vi "avoidDisturbAttackerShoot.vi"(1 "CalculatedFollowAttackerPosition":dbl[](array[numeric]), 4 "AttackingOurSelves":bool=TRUE, 5 "Game":refnum<class "Game.lvclass">, 6 "FollowAttackerPosition(FA)":dbl[](array[numeric]), 7 "field_length":i32, 8 "error in (no error)":errorcluster, 9 "AttackerPosition(AT)":dbl[](array[numeric]), 10 "Yball":dbl, 11 "FollowAttackerSkill in":refnum<class "FollowAttackerSkill.lvclass">) -> (0 "error out":errorcluster, 2 "FollowAttackerCorrectedPosition":dbl[](array[numeric]), 3 "FollowAttackerSkill out":refnum<class "FollowAttackerSkill.lvclass">)   [LabVIEW 2020, in "FollowAttackerSkill.lvclass"]
uses:
  FollowAttackerSkill.lvclass
  Game_class/Game.lvclass
  Game_class/Game.lvclass/Game.ctl
  Game_class/Read FieldRef.vi
  Game_class/Read Utilities.lvclass.vi
  Field_class/Field.lvclass
  Utilities_class/Utilities.lvclass
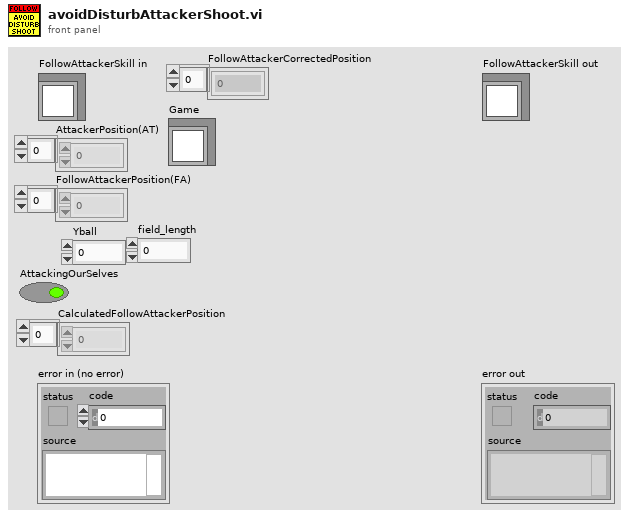
[diagram p1: front panel]
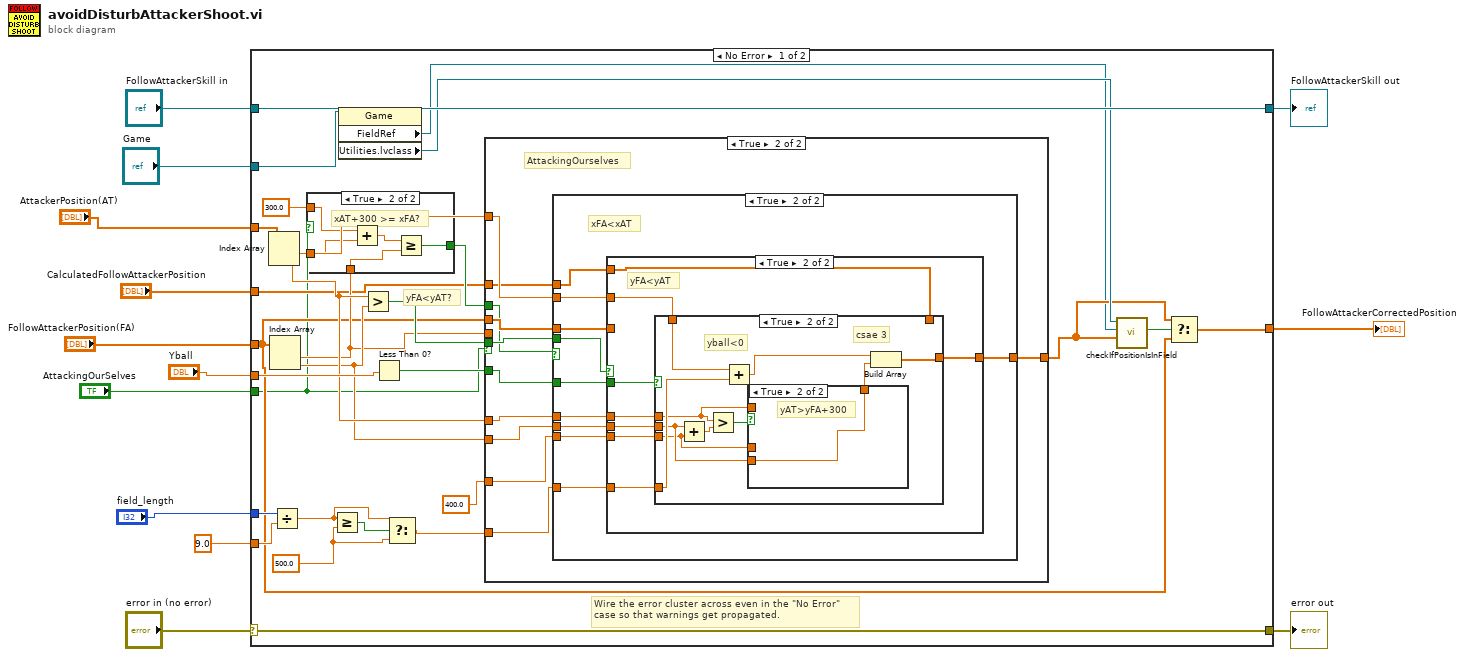
[diagram p0: block diagram]
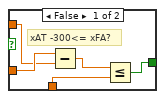
[diagram p2: hidden frame]
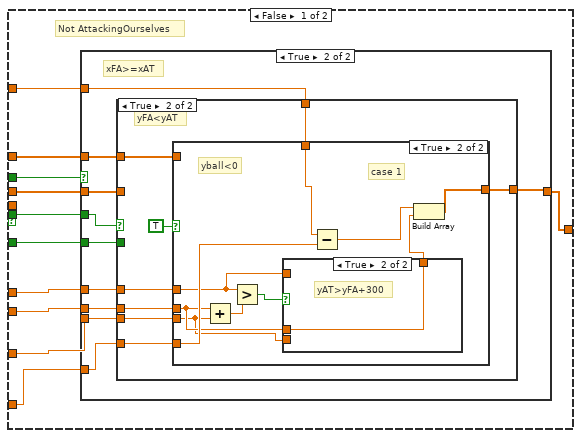
[diagram p3: hidden frame]
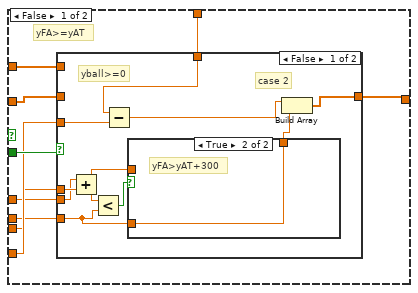
[diagram p5: hidden frame]
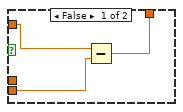
[diagram p9: hidden frame]
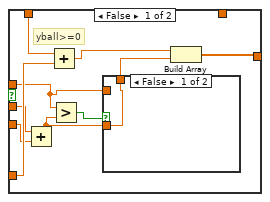
[diagram p12: hidden frame]
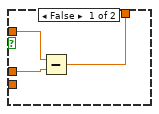
[diagram p15: hidden frame]
diagram:
  n1 = case shown="No Error" "error in (no error)" {
    selector: "error in (no error)" -> [w40 w186]
    tunnel: [w40 w186] -> w12
    tunnel: [w41 w185] -> w10
    tunnel: "FollowAttackerSkill in" -> [w41 w185]
    tunnel: "AttackingOurSelves" -> [w15 _]
    tunnel: "FollowAttackerPosition(FA)" -> [w23 _]
    tunnel: "AttackerPosition(AT)" -> [w39 _]
    tunnel: "Yball" -> [w38 _]
    tunnel: "field_length" -> [w37 _]
    tunnel: 9.0 -> [w36 _]
    tunnel: "Game" -> [w27 _]
    tunnel: [w22 _] -> w2
    tunnel: "CalculatedFollowAttackerPosition" -> [w21 _]
    frame No Error {
      w18 = 500.0 ("element")
      # "yFA<yAT?"
      # "Wire the error cluster across even in the \"No Error\"\ncase so that warnings get propagated."
      n2 = Index Array(array=w39) -> (element #1=w32:dbl, element #2=w31:dbl)  [unwired: 2 in]
      n3 = Index Array(array=w23) -> (element #1=w28:dbl, element #2=w29:dbl)  [unwired: 2 in]
      n4 = Divide(x=w37, y=w36) -> (x/y=w19:dbl)
      n5 = case shown="True" w15 {
        tunnel: [w46 w48] -> w35
        tunnel: w32 -> [w44 w51]
        tunnel: w28 -> [w45 w47]
        tunnel: 300.0 ("y") -> [w42 w50]
        frame False {
          # "xAT -300<= xFA?"
          n6 = Subtract(x=w44, y=w42) -> (x-y=w43:dbl)
          n7 = Less Or Equal?(x=w43, y=w45) -> (x <= y?=w46:bool)
        }
        frame True {
          # "xAT+300 >= xFA?"
          n8 = Add(x=w50, y=w51) -> (x+y=w49:dbl)
          n9 = Greater Or Equal?(x=w49, y=w47) -> (x >= y?=w48:bool)
        }
      }
      n10 = Greater Or Equal?(x=w19, y=w18) -> (x >= y?=w20:bool)
      n11 = property class="Game"(reference=w27) -> ("FieldRef"=w16:refnum<class "Field.lvclass">, "Utilities.lvclass"=w26:refnum<class "Utilities.lvclass">)  [unwired: 1 in, 2 out]
      n12 = Greater?(x=w31, y=w29) -> (0:w34:bool)
      n13 = Less Than 0?(x=w38) -> (x < 0?=w33:bool)
      n14 = Select(t=w19, s=w20, f=w18) -> (s? t:f=w17:dbl)
      n15 = case shown="True" w15 {
        tunnel: w17 -> [w62 w125]
        tunnel: w35 -> [w61 w119]
        tunnel: w34 -> [w60 w129]
        tunnel: w33 -> [w59 w128]
        tunnel: w32 -> [w58 w126]
        tunnel: w31 -> [w57 w122]
        tunnel: 400.0 -> [w56 w124]
        tunnel: w29 -> [w55 w123]
        tunnel: w23 -> [w54 w127]
        tunnel: w28 -> [_ _]
        tunnel: [w53 w121] -> w24
        tunnel: w21 -> [w52 w120]
        frame False {
          # "Not AttackingOurselves"
          n16 = case shown="True" w61 {
            tunnel: w62 -> [_ w70]
            tunnel: w60 -> [_ w73]
            tunnel: w59 -> [_ w72]
            tunnel: w58 -> [_ w71]
            tunnel: w57 -> [_ w69]
            tunnel: w56 -> [_ w68]
            tunnel: w55 -> [_ w67]
            tunnel: w54 -> [_ w66]
            tunnel: [w63 w65] -> w53
            tunnel: w52 -> [w63 w64]
            frame False {
            }
            frame True {
              # "xFA>=xAT"
              n17 = case shown="True" w73 {
                tunnel: w72 -> [w82 _]
                tunnel: w71 -> [w81 w103]
                tunnel: w70 -> [w80 w102]
                tunnel: w69 -> [w78 w101]
                tunnel: w68 -> [w79 w100]
                tunnel: w67 -> [w77 w99]
                tunnel: w66 -> [w76 _]
                tunnel: [w75 w98] -> w65
                tunnel: w64 -> [w74 w97]
                frame False {
                  # "yFA>=yAT"
                  n18 = case shown="False" w82 {
                    tunnel: w81 -> [w92 _]
                    tunnel: w80 -> [w91 _]
                    tunnel: w79 -> [w90 _]
                    tunnel: w78 -> [w89 _]
                    tunnel: w77 -> [w87 _]
                    tunnel: [w83 w95] -> w75
                    tunnel: w76 -> [_ _]
                    tunnel: w74 -> [_ w95]
                    frame False {
                      # "case 2"
                      # "yball>=0"
                      n19 = Add(x=w89, y=w90) -> (x+y=w86:dbl)
                      n20 = Less?(x=w86, y=w87) -> (x < y?=w88:bool)
                      n21 = Subtract(x=w92, y=w91) -> (x-y=w85:dbl)
                      n22 = case shown="True" w88 {
                        tunnel: [w93 w94] -> w84
                        tunnel: w87 -> [_ w94]
                        tunnel: w86 -> [w93 _]
                        frame False {
                        }
                        frame True {
                          # "yFA>yAT+300"
                        }
                      }
                      n23 = Build Array(w85, w84) -> (w83:dbl[])
                    }
                    frame True {
                    }
                  }
                }
                frame True {
                  # "yFA<yAT"
                  n24 = case shown="True" TRUE {
                    tunnel: w103 -> [_ w114]
                    tunnel: w102 -> [_ w113]
                    tunnel: w101 -> [_ w108]
                    tunnel: w100 -> [_ w109]
                    tunnel: w99 -> [_ w110]
                    tunnel: [w104 w105] -> w98
                    tunnel: w97 -> [w104 _]
                    frame False {
                    }
                    frame True {
                      # "case 1"
                      # "yball<0"
                      n25 = Add(x=w110, y=w109) -> (x+y=w111:dbl)
                      n26 = Greater?(x=w108, y=w111) -> (0:w112:bool)
                      n27 = case shown="True" w112 {
                        tunnel: [w115 w118] -> w106
                        tunnel: w110 -> [_ w118]
                        tunnel: w109 -> [w117 _]
                        tunnel: w108 -> [w116 _]
                        frame False {
                          n28 = Subtract(x=w116, y=w117) -> (x-y=w115:dbl)
                        }
                        frame True {
                          # "yAT>yFA+300"
                        }
                      }
                      n29 = Subtract(x=w114, y=w113) -> (x-y=w107:dbl)
                      n30 = Build Array(w107, w106) -> (w105:dbl[])
                    }
                  }
                }
              }
            }
          }
        }
        frame True {
          # "AttackingOurselves"
          n31 = case shown="True" w119 {
            tunnel: w129 -> [_ w140]
            tunnel: w128 -> [_ w139]
            tunnel: w127 -> [_ w138]
            tunnel: w126 -> [_ w137]
            tunnel: w125 -> [_ w136]
            tunnel: w124 -> [_ w135]
            tunnel: w123 -> [_ w134]
            tunnel: w122 -> [_ w133]
            tunnel: [w130 w132] -> w121
            tunnel: w120 -> [w130 w131]
            frame False {
            }
            frame True {
              # "xFA<xAT"
              n32 = case shown="True" w140 {
                tunnel: w139 -> [w148 w169]
                tunnel: w138 -> [_ _]
                tunnel: w137 -> [w145 w168]
                tunnel: w136 -> [w146 w167]
                tunnel: w135 -> [w144 w166]
                tunnel: w134 -> [w142 w165]
                tunnel: w133 -> [w143 w164]
                tunnel: [w147 w163] -> w132
                tunnel: w131 -> [w141 w162]
                frame False {
                  # "yFA>=yAT"
                  n33 = case shown="True" w148 {
                    tunnel: [w155 w161] -> w147
                    tunnel: w146 -> [w158 _]
                    tunnel: w145 -> [w157 _]
                    tunnel: w144 -> [w154 _]
                    tunnel: w143 -> [w153 _]
                    tunnel: w142 -> [w150 _]
                    tunnel: w141 -> [_ w161]
                    frame False {
                      # "yball>=0"
                      n34 = Add(x=w153, y=w154) -> (x+y=w149:dbl)
                      n35 = Add(x=w157, y=w158) -> (x+y=w156:dbl)
                      n36 = Greater?(x=w150, y=w149) -> (0:w152:bool)
                      n37 = case shown="False" w152 {
                        tunnel: [w159 w160] -> w151
                        tunnel: w150 -> [_ w160]
                        tunnel: w149 -> [w159 _]
                        frame False {
                        }
                        frame True {
                          # "yFA>yAT+300"
                        }
                      }
                      n38 = Build Array(w156, w151) -> (w155:dbl[])
                    }
                    frame True {
                    }
                  }
                }
                frame True {
                  # "yFA<yAT"
                  n39 = case shown="True" w169 {
                    tunnel: [w170 w176] -> w163
                    tunnel: w168 -> [_ w180]
                    tunnel: w167 -> [_ w179]
                    tunnel: w166 -> [_ w172]
                    tunnel: w165 -> [_ w173]
                    tunnel: w164 -> [_ w171]
                    tunnel: w162 -> [w170 _]
                    frame False {
                    }
                    frame True {
                      # "csae 3"
                      # "yball<0"
                      n40 = Add(x=w173, y=w172) -> (x+y=w177:dbl)
                      n41 = Greater?(x=w171, y=w177) -> (0:w178:bool)
                      n42 = Add(x=w180, y=w179) -> (x+y=w175:dbl)
                      n43 = case shown="True" w178 {
                        tunnel: [w181 w184] -> w174
                        tunnel: w173 -> [_ w184]
                        tunnel: w172 -> [w183 _]
                        tunnel: w171 -> [w182 _]
                        frame False {
                          n44 = Subtract(x=w182, y=w183) -> (x-y=w181:dbl)
                        }
                        frame True {
                          # "yAT>yFA+300"
                        }
                      }
                      n45 = Build Array(w175, w174) -> (w176:dbl[])
                    }
                  }
                }
              }
            }
          }
        }
      }
      n46 = call "checkIfPositionIsInField.vi"("Position"=w24, "FieldRef"=w16, "Utilities in"=w26) -> ("Position Is In Field?"=w25:bool)  [unwired: 4 in, 4 out]
      n47 = Select(t=w24, s=w25, f=w23) -> (s? t:f=w22:dbl[])
    }
    frame Error {
    }
  }
  "error out" <- w12
  "FollowAttackerSkill out" <- w10
  "FollowAttackerCorrectedPosition" <- w2
